vi "R2R-Controller-PCTesting.vi"() -> ()   [LabVIEW 2013]
uses:
  controls/Control Configuration.ctl
  controls/Custom Controller Inputs.ctl
  <vilib>/rvi/Analysis/measure/butterworth/XNode/niFpgaButterworthFilter.xnode
  <vilib>/addons/control/pid/fpga.llb/XNode/niFpgaPID.xnode
panel:
  out "PWM Duty Cycle":i16
  out "V*(V)":fxp<+/-,53,13> format="%.6f"
  out "Y*'":fxp<+/-,36,35>
  out "X(mm)":fxp<+/-,35,12>
  out "Y*":fxp<+/-,64,31>
  out "Duty Cycle Output":i16
  in  "K_PosSense (mm/Volt)":fxp<+,12,4>=10.0
  out "DeltaX*":fxp<+/-,32,11>
  in  "Reset Integrator":bool
  out "F_Error (N)":fxp<+/-,40,11>
  in  "K_PWM (Counts/Volt)":fxp<+,16,7>=83.33203125
  in  "Ra (Armature Resistance) (Ohms)":fxp<+/-,7,7>=60.0
  in  "Custom Controller Inputs":T1
  in  "X (Raw Analog V)":fxp<+,18,3>
  in  "F (Raw Analog V)":fxp<+,18,3>
  in  "X* (mm)":fxp<+/-,16,7>
  in  "F* (N)":fxp<+/-,16,7>
  in  "Gain Configuration":T2={"PID Gains"={"proportional gain (Kc)"=1.0, "integral gain (Kc*Ts/Ti)"=0.0, "derivative gain (Kc*Td/Ts)"=0.0}, "Output Range"={"output high"=10.0, "output low"=-10.0}}
  out "I* Current Command (A)":fxp<+/-,48,8>
  out "Measured Force (N)":fxp<+,39,10>
  in  "Force Sensor Gain (N/V)":fxp<+,20,6>=53.02703857421875
  in  "L12 Gain (mA/N)":fxp<+,16,2>=2.29180908203125
  in  "L12 Offset (mA)":fxp<+,18,4>=12.9949951171875
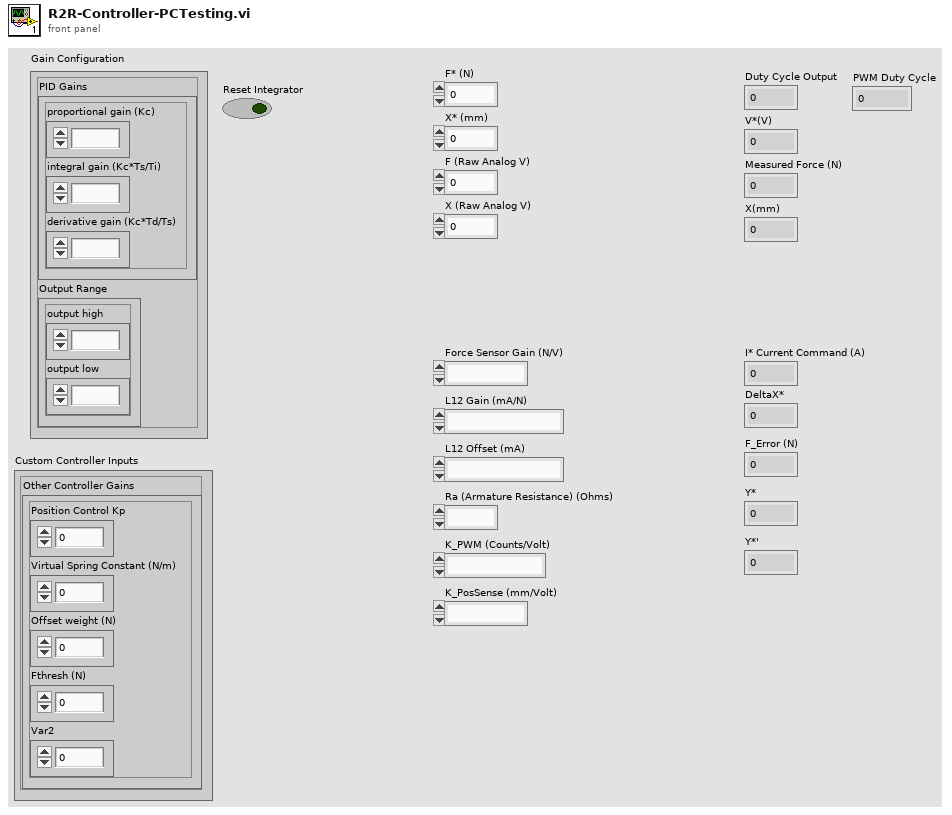
[diagram p1: front panel]
types:
  T1 = typedef "Custom Controller Inputs.ctl" = cluster{"Other Controller Gains":cluster{"Position Control Kp":fxp<+/-,16,8>, "Virtual Spring Constant (N/m)":fxp<+,16,12>, "Offset weight (N)":fxp<+/-,16,8>, "Fthresh (N)":fxp<+/-,16,5>, "Var2":fxp<+/-,16,5>}}
  T2 = typedef "Control Configuration.ctl" = cluster{"PID Gains":cluster{"proportional gain (Kc)":fxp<+/-,16,8>, "integral gain (Kc*Ts/Ti)":fxp<+/-,16,8>, "derivative gain (Kc*Td/Ts)":fxp<+/-,16,8>}, "Output Range":cluster{"output high":fxp<+/-,16,7>, "output low":fxp<+/-,16,7>}}
  T3 = cluster{"Position Control Kp":fxp<+/-,16,8>, "Virtual Spring Constant (N/m)":fxp<+,16,12>, "Offset weight (N)":fxp<+/-,16,8>, "Fthresh (N)":fxp<+/-,16,5>, "Var2":fxp<+/-,16,5>}
  T4 = cluster{"proportional gain (Kc)":fxp<+/-,16,8>, "integral gain (Kc*Ts/Ti)":fxp<+/-,16,8>, "derivative gain (Kc*Td/Ts)":fxp<+/-,16,8>}
  T5 = cluster{"output high":fxp<+/-,16,7>, "output low":fxp<+/-,16,7>}
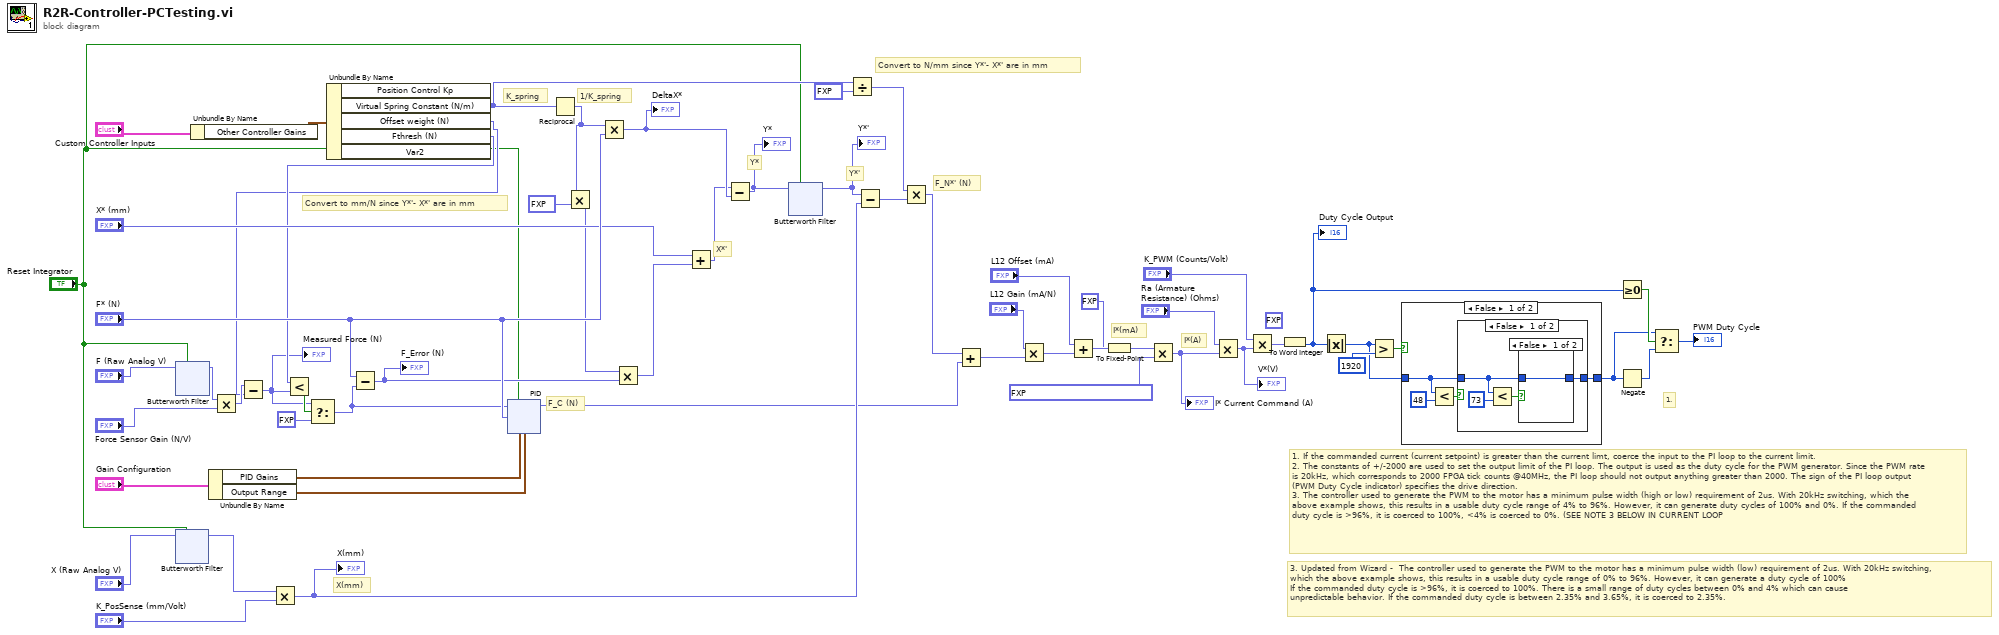
[diagram p0: block diagram]
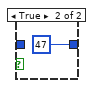
[diagram p2: hidden frame]
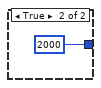
[diagram p4: hidden frame]
diagram:
  (unwired) fxp<+/-,16,16> 0.0 ("fixed-point type")
  # "Convert to mm/N since Y*'- X*' are in mm"
  # "Convert to N/mm since Y*'- X*' are in mm"
  # "1. If the commanded current (current setpoint) is greater than the current limt, coerce the input to the PI loop to the current limit.\n2. The constants of +/-2000 are used to set the output limit of the PI loop. The output is used as the duty cycle for the PWM generator. Since the PWM rate is 20kHz, which corresponds to 2000 FPGA tick counts @40MHz, the PI loop should not output anything greater than 2000. The sign of the PI loop output (PWM Duty Cycle indicator) specifies the drive direction.\n3. The controller used to generate the PWM to the motor has a minimum pulse width (high or low) requirement of 2us. With 20kHz switching, which the above example shows, this results in a usable duty cycle range of 4% to 96%. However, it can generate duty cycles of 100% and 0%. If the commanded duty cycle is >96%, it is coerced to 100%, <4% is coerced to 0%. (SEE NOTE 3 BELOW IN CURRENT LOOP"
  # "3. Updated from Wizard -  The controller used to generate the PWM to the motor has a minimum pulse width (low) requirement of 2us. With 20kHz switching, which the above example shows, this results in a usable duty cycle range of 0% to 96%. However, it can generate a duty cycle of 100%\nIf the commanded duty cycle is >96%, it is coerced to 100%. There is a small range of duty cycles between 0% and 4% which can cause\nunpredictable behavior. If the commanded duty cycle is between 2.35% and 3.65%, it is coerced to 2.35%."
  # "1."
  # "Y*'"
  # "I*(A)"
  # "I*(mA)"
  # "F_C (N)"
  # "F_N*' (N)"
  # "X(mm)"
  # "Y*"
  # "X*'"
  # "K_spring"
  # "1/K_spring"
  n1 = xnode "Butterworth Filter"("input data"="X (Raw Analog V)", "reset"="Reset Integrator") -> ("output data"=w2:fxp<+/-,23,8>)  [unwired: 1 in]
  n2 = xnode "Butterworth Filter"("input data"="F (Raw Analog V)", "reset"="Reset Integrator") -> ("output data"=w5:fxp<+/-,23,8>)  [unwired: 1 in]
  n3 = Unbundle By Name("Custom Controller Inputs") -> ("Other Controller Gains"=w53:T3)
  n4 = Unbundle By Name("Gain Configuration") -> ("PID Gains"=w57:T4, "Output Range"=w56:T5)
  n5 = Multiply(x=w5, y="Force Sensor Gain (N/V)") -> (x*y=w8:fxp<+/-,43,14>)
  n6 = Multiply(x=w2, y="K_PosSense (mm/Volt)") -> (x*y=w44:fxp<+/-,35,12>)
  "X(mm)" <- w44
  n7 = Unbundle By Name(w53) -> ("Virtual Spring Constant (N/m)"=w42:fxp<+,16,12>, "Offset weight (N)"=w7:fxp<+/-,16,8>, "Fthresh (N)"=w9:fxp<+/-,16,5>)  [unwired: 2 out]
  n8 = Subtract(x=w8, y=w7) -> (x-y=w6:fxp<+/-,44,15>)
  "Measured Force (N)" <- w6
  n9 = Less?(x=w9, y=w6) -> (x < y?=w15:bool)
  n10 = Select(t=w6, s=w15, f=fxp<+,38,9> 0.0) -> (s? t:f=w13:fxp<+/-,44,15>)
  n11 = Subtract(x="F* (N)", y=w13) -> (x-y=w51:fxp<+/-,44,15>)
  "F_Error (N)" <- w51
  n12 = xnode "PID"("process variable"=w13, "reset?"="Reset Integrator", "setpoint"="F* (N)", "PID gains"=w57, "output range"=w56) -> ("output"=w40:fxp<+/-,16,15>)
  n13 = Reciprocal(x=w42) -> (1/x=w50:fxp<+,17,5>)
  n14 = Multiply(x=w50, y=fxp<+,17,10> 1000.0) -> (x*y=w20:fxp<+,33,14>)
  n15 = Multiply(x=w50, y="F* (N)") -> (x*y=w47:fxp<+/-,32,11>)
  "DeltaX*" <- w47
  n16 = Multiply(x=w20, y=w51) -> (x*y=w48:fxp<+/-,64,29>)
  n17 = Add(x="X* (mm)", y=w48) -> (x+y=w46:fxp<+/-,64,30>)
  n18 = Subtract(x=w46, y=w47) -> (x-y=w31:fxp<+/-,64,31>)
  "Y*" <- w31
  n19 = xnode "Butterworth Filter"("input data"=w31, "reset"="Reset Integrator") -> ("output data"=w30:fxp<+/-,36,35>)  [unwired: 1 in]
  "Y*'" <- w30
  n20 = Divide(x=w42, y=fxp<+,16,12> 1000.0) -> (x/y=w22:fxp<+,32,16>)
  n21 = Subtract(x=w30, y=w44) -> (x-y=w43:fxp<+/-,59,36>)
  n22 = Multiply(x=w22, y=w43) -> (x*y=w41:fxp<+/-,64,51>)
  n23 = Add(x=w41, y=w40) -> (x+y=w38:fxp<+/-,64,52>)
  n24 = Multiply(x="L12 Gain (mA/N)", y=w38) -> (x*y=w37:fxp<+/-,64,54>)
  n25 = Add(x="L12 Offset (mA)", y=w37) -> (x+y=w18:fxp<+/-,64,55>)
  n26 = To Fixed-Point(fixed-point type=fxp<+/-,32,16> 0.0, number=w18) -> (fixed-point=w16:fxp<+/-,32,16>)
  n27 = Multiply(x=w16, y=fxp<+/-,16,-8> 0.0009999871253967285) -> (x*y=w10:fxp<+/-,48,8>)
  "I* Current Command (A)" <- w10
  n28 = Multiply(x="Ra (Armature Resistance) (Ohms)", y=w10) -> (x*y=w33:fxp<+/-,53,13>)
  "V*(V)" <- w33
  n29 = Multiply(x="K_PWM (Counts/Volt)", y=w33) -> (x*y=w12:fxp<+/-,64,20>)
  n30 = To Word Integer(number=w12) -> (16bit integer=w11:i16)
  "Duty Cycle Output" <- w11
  n31 = Absolute Value(x=w11) -> (abs(x)=w24:i16)
  n32 = Greater?(x=w24, y=i16 1920 ("upper limit")) -> (0:w26:bool)
  n33 = case shown="False" w26 {
    tunnel: [w61 i16 2000 ("upper limit")] -> w25
    tunnel: w24 -> [w59 _]
    frame False {
      n34 = Less?(x=w59, y=i16 48 ("lower limit")) -> (x < y?=w60:bool)
      n35 = case shown="False" w60 {
        tunnel: [w63 w69] -> w61
        tunnel: w59 -> [w64 w69]
        frame False {
          n36 = Less?(x=w64, y=i16 73 ("lower limit")) -> (x < y?=w65:bool)
          n37 = case shown="False" w65 {
            tunnel: w64 -> [w67 _]
            tunnel: [w67 i16 47 ("lower limit")] -> w63
            frame False {
            }
            frame True {
            }
          }
        }
        frame True {
        }
      }
    }
    frame True {
    }
  }
  n38 = Greater Or Equal To 0?(x=w11) -> (x >= 0?=w29:bool)
  n39 = Negate(x=w25) -> (-x=w28:i16)
  n40 = Select(t=w25, s=w29, f=w28) -> (s? t:f=→"PWM Duty Cycle":i16)
